vi "ConfigureTestPanel.vi"(8 "error in (no error)":errorcluster) -> (0 "error out":errorcluster, 3 "Test Panel Config out":T1)   [LabVIEW 2017, in "CmsTestPanel.lvlib"]
uses:
  <vilib>/addons/InsightCM/Devices/Shared/Cms/CmsTestPanel/CmsTestPanel.lvlib
  <vilib>/addons/InsightCM/Devices/Shared/Cms/CmsTestPanel/controls/Configuration.ctl
  <vilib>/addons/InsightCM/Devices/Shared/Common/TestPanel/controls/Configuration.ctl
  <vilib>/addons/InsightCM/Devices/Shared/Common/TestPanel/controls/State.ctl
  <vilib>/addons/InsightCM/MessageBus/Base/controls/IRoutingSource.ctl
  <vilib>/addons/InsightCM/MessageBus/Base/controls/TestPanelTimeSeries.ctl
  <vilib>/addons/InsightCM/MessageBus/Base/controls/TestPanelValue.ctl
  <vilib>/addons/InsightCM/Utilities/GlobalConfiguration/GlobalConfiguration.lvlib
  <vilib>/addons/InsightCM/Utilities/DeviceModelHelpers/DeviceModelHelpers.lvlib
  <vilib>/addons/InsightCM/Utilities/PropertyHelpers/PropertyHelpers.lvlib
  <vilib>/addons/InsightCM/Devices/Shared/Common/TestPanel/TestPanel.lvlib
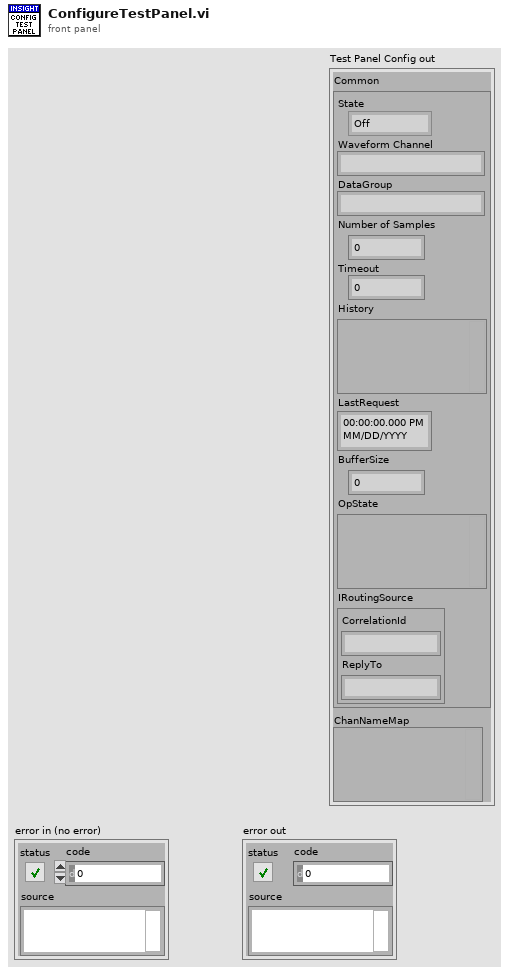
[diagram p1: front panel]
types:
  T1 = typedef "CmsTestPanel.lvlib/Configuration.ctl" = cluster{"Common":T2, "ChanNameMap":variant}
  T2 = typedef "TestPanel.lvlib/Configuration.ctl" = cluster{"State":T3, "Waveform Channel":string, "DataGroup":string, "Number of Samples":i32, "Timeout":dbl, "History":variant, "LastRequest":timestamp, "BufferSize":i32, "OpState":variant, "IRoutingSource":T4}
  T3 = typedef "TestPanel.lvlib/State.ctl" = enum16{"Off", "On", "PendingValues", "PendingDataSet"}
  T4 = typedef "IRoutingSource.ctl" = cluster{"CorrelationId":string, "ReplyTo":string}
  T5 = typedef "SectionKeyValues.ctl" = cluster{"Section":string, "KeyValues":T6[]}
  T6 = typedef "KeyValuePair.ctl" = cluster{"Key":string, "Value":string}
  T7 = typedef "R2_DeviceModel.ctl" = cluster{"Device":T8, "Channels":T15[], "Tags":T17[]}
  T8 = typedef "R2_Device.ctl" = cluster{"Id":string, "Name":string, "DeviceType":string, "HardwareName":string, "IpAddress":string, "HardwareInfo":T6[], "ApplicationType":string, "ApplicationVersion":string, "EquipmentIds":string[], "ConfigurationVersion":string, "State":T9, "Properties":T6[], "DataGroups":T10[], "BurstModeTrigger":T14}
  T9 = typedef "DeviceState.ctl" = cluster{"Disabled":bool}
  T10 = typedef "R2_DataGroup.ctl" = cluster{"Name":string, "OperatingStates":T11[], "Properties":T6[], "EquipmentIds":string[], "AssetNodeId":string}
  T11 = typedef "OperatingState.ctl" = cluster{"Name":string, "Properties":T6[], "Triggers":T12[]}
  T12 = typedef "Trigger.ctl" = cluster{"Type":string, "Expression":string, "Conditions":T13[]}
  T13 = typedef "Condition.ctl" = cluster{"Source":string, "Type":string, "Operator":string, "CompareTo":string, "DwellSeconds":dbl}
  T14 = typedef "BurstModeTrigger.ctl" = cluster{"Trigger":T12, "SampleRate":string, "AcquisitionLength":string}
  T15 = typedef "R2_Channel.ctl" = cluster{"Id":string, "DeviceId":string, "Name":string, "ChannelType":string, "HardwareKey":string, "HardwareChannel":string, "DataGroup":string, "Keywords":string[], "EquipmentIds":string[], "Properties":T6[], "Metrics":T16[], "AssetNodeId":string, "MeasType":string, "AssetName":string}
  T16 = typedef "Metric.ctl" = cluster{"Id":string, "Name":string, "Unit":string, "Properties":T6[], "MetricDefinitionInstanceId":string}
  T17 = typedef "Tag.ctl" = cluster{"Id":string, "Path":string, "Name":string, "Datatype":string, "Props":T6[], "Keywords":string[]}
  T18 = typedef "AssetNode.ctl" = cluster{"Id":string, "Type":string, "Name":string, "ParentIds":string[], "State":T19, "MeasType":string, "Properties":T6[], "OperatingStates":T11[], "Metrics":T16[], "TrendAlarmRules":T20[], "References":T23[]}
  T19 = typedef "AssetState.ctl" = cluster{"Disabled":bool}
  T20 = typedef "TrendAlarmRule.ctl" = cluster{"Id":string, "AssetNodeId":string, "TrendId":string, "Disabled":bool, "OperatingState":string, "Operator":string, "Hysteresis":dbl, "OnDelaySeconds":dbl, "OffDelaySeconds":dbl, "Levels":T21[], "Properties":T6[]}
  T21 = typedef "TrendAlarmLevel.ctl" = cluster{"Severity":i32, "CompareTo":dbl, "Actions":T22[]}
  T22 = typedef "AlarmAction.ctl" = cluster{"Type":string, "Props":T6[]}
  T23 = typedef "AssetNodeReference.ctl" = cluster{"NodeId":string, "Name":string}
  T24 = typedef "TestPanelTimeSeries.ctl" = cluster{"TrendPointId":string, "AssetName":string, "MetricName":string, "Unit":string, "Values":T25[]}
  T25 = typedef "TestPanelValue.ctl" = cluster{"Value":dbl, "Timestamp":i64, "Invalid":bool}
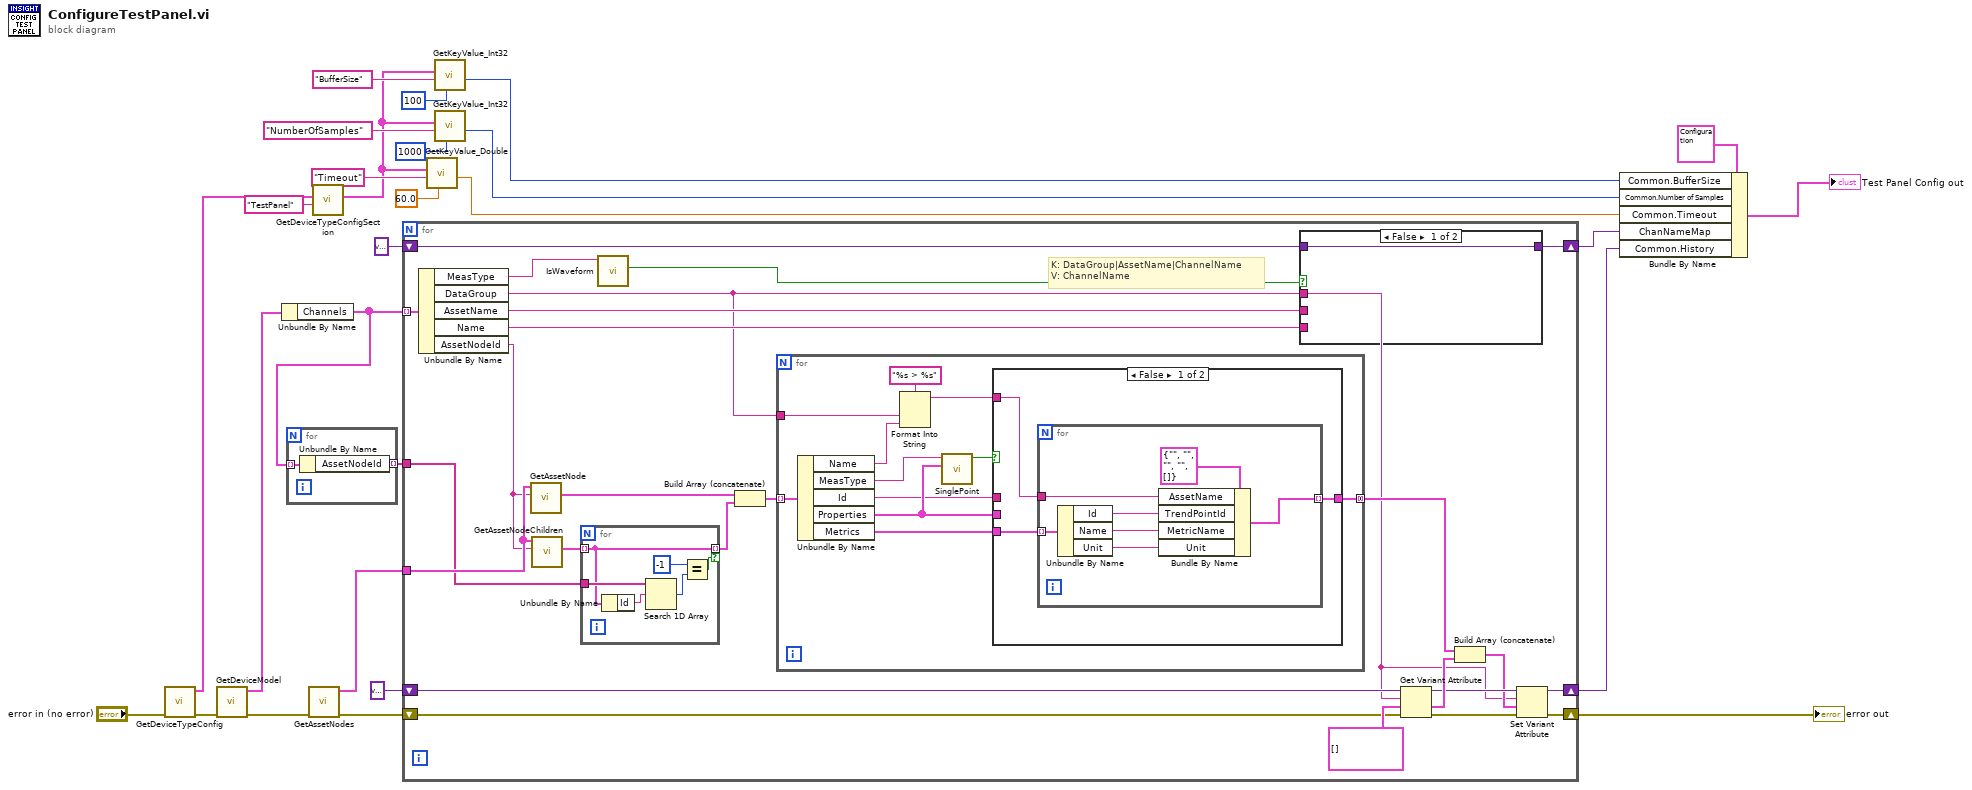
[diagram p0: block diagram]
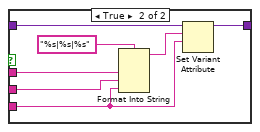
[diagram p2: hidden frame]
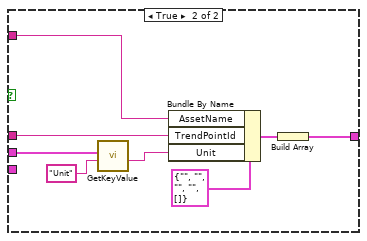
[diagram p3: hidden frame]
diagram:
  n1 = call <vilib>:"GetDeviceTypeConfig.vi"("error in (no error)"="error in (no error)") -> ("error out"=w10:errorcluster, "key values"=w22:T5[])  [unwired: 8 in, 1 out]
  n2 = call <vilib>:"GetDeviceModel.vi"("error in (no error)"=w10) -> ("error out"=w11:errorcluster, "device model"=w25:T7)  [unwired: 8 in, 1 out]
  n3 = Unbundle By Name(w25) -> ("Channels"=w4:T15[])
  n4 = for {
    tunnel: w4 -> [w29] mode=indexing
    tunnel: [w28] -> w3 mode=indexing
    n5 = Unbundle By Name(w29) -> ("AssetNodeId"=w28:string)
  }
  n6 = call <vilib>:"GetAssetNodes.vi"("error in (no error)"=w11) -> ("error out"=w12:errorcluster, "AssetNodes"=w24:T18[])  [unwired: 8 in, 1 out]
  n7 = call <vilib>:"GetDeviceTypeConfigSection.vi"("key"="TestPanel", "key values"=w22) -> ("key value pairs out"=w7:T6[])  [unwired: 8 in, 1 out]
  n8 = for {
    tunnel: w4 -> [w35] mode=indexing
    tunnel: w24 -> [w54]
    shift-right: [w44] -> w14
    shift-left: variant -> [w50]
    shift-right: [w42] -> w13
    shift-left: w12 -> [w41]
    tunnel: w3 -> [w39]
    shift-right: [w36] -> w1
    shift-left: variant -> [w37]
    # "K: DataGroup|AssetName|ChannelName\nV: ChannelName"
    n9 = Unbundle By Name(w35) -> ("MeasType"=w32:string, "DataGroup"=w30:string, "AssetName"=w34:string, "Name"=w33:string, "AssetNodeId"=w53:string)
    n10 = call <vilib>:"GetAssetNode.vi"("node id"=w53, "nodes in"=w54) -> ("AssetNode"=w52:T18)  [unwired: 7 in, 2 out]
    n11 = call <vilib>:"GetAssetNodeChildren.vi"("node id"=w53, "nodes in"=w54) -> ("Children"=w40:T18[])  [unwired: 8 in, 1 out]
    n12 = for {
      tunnel: w40 -> [w65] mode=indexing
      tunnel: w39 -> [w67]
      tunnel: [w65] -> w38 mode=indexing if=w63
      n13 = Unbundle By Name(w65) -> ("Id"=w68:string)
      n14 = Search 1D Array(1D array=w67, element=w68) -> (index of element=w66:i32)  [unwired: 1 in]
      n15 = Equal?(x=-1, y=w66) -> (x = y?=w63:bool)
    }
    n16 = call <vilib>:"IsWaveform.vi"("MeasType"=w32) -> ("is waveform"=w31:bool)  [unwired: 10 in]
    n17 = Build Array (concatenate)(w52, w38) -> (w51:T18[])
    n18 = for {
      tunnel: w51 -> [w79] mode=indexing
      tunnel: [w77] -> w47 mode=concatenating
      tunnel: w30 -> [w74]
      n19 = Unbundle By Name(w79) -> ("Name"=w73:string, "MeasType"=w71:string, "Id"=w69:string, "Properties"=w70:T6[], "Metrics"=w78:T16[])
      n20 = Format Into String(format string="%s > %s", w74, w73) -> (resulting string=w72:string)  [unwired: 2 in, 1 out]
      n21 = call <vilib>:"SinglePoint.vi"("Properties"=w70, "MeasType"=w71) -> ("Single Point"=w76:bool)  [unwired: 9 in]
      n22 = case shown="False" w76 {
        tunnel: w69 -> [_ w96]
        tunnel: [w81 w94] -> w77
        tunnel: w78 -> [w82 _]
        tunnel: w70 -> [_ w92]
        tunnel: w72 -> [w80 w90]
        frame False {
          n23 = for {
            tunnel: w82 -> [w88] mode=indexing
            tunnel: [w86] -> w81 mode=indexing
            tunnel: w80 -> [w85]
            n24 = Unbundle By Name(w88) -> ("Id"=w87:string, "Name"=w84:string, "Unit"=w83:string)
            n25 = Bundle By Name(cluster=T24 {"TrendPointId"="", "AssetName"="", "MetricName"="", "Unit"="", "Values"=[]} ("History"), "AssetName"=w85, "TrendPointId"=w87, "MetricName"=w84, "Unit"=w83) -> (w86:T24)
          }
        }
        frame True {
          n26 = call <vilib>:"GetKeyValue.vi"("key"="Unit" ("name"), "key value pairs"=w92) -> ("value"=w91:string)  [unwired: 7 in, 2 out]
          n27 = Bundle By Name(cluster=T24 {"TrendPointId"="", "AssetName"="", "MetricName"="", "Unit"="", "Values"=[]} ("History"), "AssetName"=w90, "TrendPointId"=w96, "Unit"=w91) -> (w95:T24)
          n28 = Build Array(w95) -> (w94:T24[])
        }
      }
    }
    n29 = case shown="False" w31 {
      tunnel: w37 -> [w55 w62]
      tunnel: [w55 w61] -> w36
      tunnel: w30 -> [_ w59]
      tunnel: w34 -> [_ w57]
      tunnel: w33 -> [_ w56]
      frame False {
      }
      frame True {
        n30 = Format Into String(format string="%s|%s|%s", w59, w57, w56) -> (resulting string=w58:string)  [unwired: 2 in, 1 out]
        n31 = Set Variant Attribute(Variant=w62, name=w58, value=w56) -> (Variant out=w61:variant)  [unwired: 1 in, 2 out]
      }
    }
    n32 = Get Variant Attribute(Variant=w50, name=w30, default value (empty Variant)=T24[] [], error in=w41) -> (duplicate Variant=w46:variant, value=w48:T24[], error out=w43:errorcluster)  [unwired: 1 out]
    n33 = Build Array (concatenate)(w47, w48) -> (w45:T24[])
    n34 = Set Variant Attribute(Variant=w46, name=w30, value=w45, error in=w43) -> (Variant out=w44:variant, error out=w42:errorcluster)  [unwired: 1 out]
  }
  "error out" <- w13
  n35 = call <vilib>:"GetKeyValue_Double.vi"("default"=60.0, "key"="Timeout", "key value pairs"=w7) -> ("value"=w16:dbl)  [unwired: 6 in, 2 out]
  n36 = call <vilib>:"GetKeyValue_Int32.vi"("default"=100, "key"="BufferSize", "key value pairs"=w7) -> ("value"=w5:i32)  [unwired: 6 in, 2 out]
  n37 = call <vilib>:"GetKeyValue_Int32.vi"("default"=1000, "key"="NumberOfSamples", "key value pairs"=w7) -> ("value"=w15:i32)  [unwired: 6 in, 2 out]
  n38 = Bundle By Name(cluster=T1 {"Common"={"State"=enum."Off", "Waveform Channel"="", "DataGroup"="", "Number of Samples"=0, "Timeout"=0.0, "History"=variant, "LastRequest"=timestamp(0 s since 1904-01-01), "BufferSize"=0, "OpState"=variant, "IRoutingSource"={"CorrelationId"="", "ReplyTo"=""}}, "ChanNameMap"=variant} ("Test Panel Config"), "Common.BufferSize"=w5, "Common.Number of Samples"=w15, "Common.Timeout"=w16, "ChanNameMap"=w1, "Common.History"=w14) -> (→"Test Panel Config out":T1)
